vi "Comunicacion_con_Leds.vi"() -> ()   [LabVIEW 2020]
panel:
  in  "Stop":bool
  out "Valor hexadecimal":dbl
  in  "Botón de Contador":bool
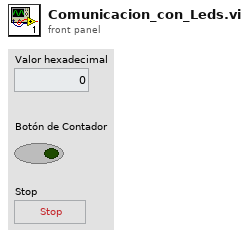
[diagram p1: front panel]
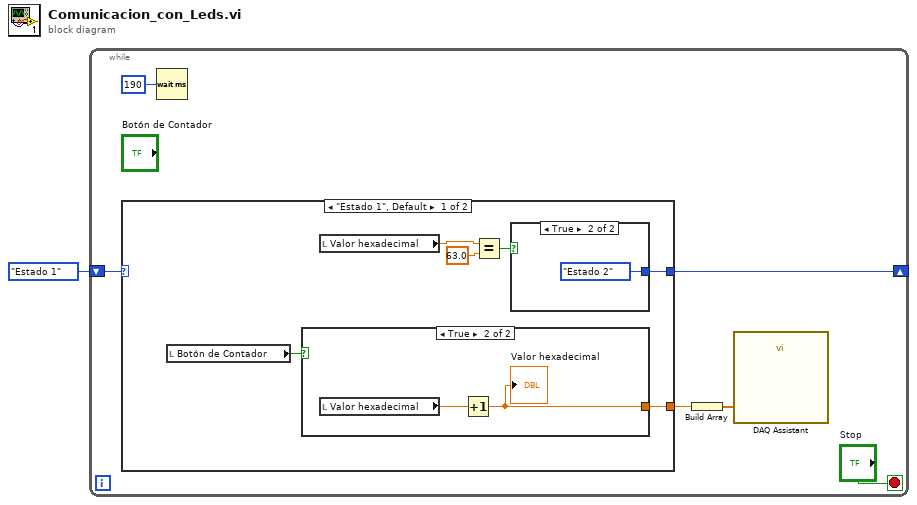
[diagram p0: block diagram]
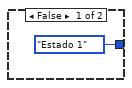
[diagram p2: hidden frame]
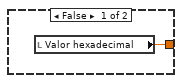
[diagram p3: hidden frame]
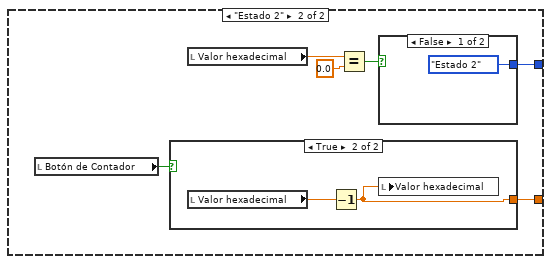
[diagram p4: hidden frame]
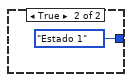
[diagram p5: hidden frame]
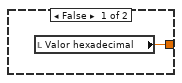
[diagram p6: hidden frame]
diagram:
  n1 = while {
    shift-right: [w5] -> _
    shift-left: enum16{"Estado 1", "Estado 2"}."Estado 1" -> [w6]
    stop <- "Stop" stop-if-true
    n2 = case shown="\"Estado 1\", Default" w6 {
      tunnel: [w13 w24] -> w5
      tunnel: [w11 w23] -> w3
      frame "Estado 1", Default {
        n3 = local read "Botón de Contador"() -> (w12:bool)
        n4 = case shown="True" w12 {
          tunnel: [w16 w18] -> w11
          frame False {
            n5 = local read "Valor hexadecimal"() -> (w16:dbl)
          }
          frame True {
            n6 = local read "Valor hexadecimal"() -> (w17:dbl)
            n7 = Increment(x=w17) -> (x+1=w18:dbl)
            "Valor hexadecimal" <- w18
          }
        }
        n8 = local read "Valor hexadecimal"() -> (w10:dbl)
        n9 = Equal?(x=w10, y=63.0) -> (x = y?=w8:bool)
        n10 = case shown="True" w8 {
          tunnel: [enum16{"Estado 1", "Estado 2"}."Estado 1" enum16{"Estado 1", "Estado 2"}."Estado 2"] -> w13
          frame False {
          }
          frame True {
          }
        }
      }
      frame "Estado 2" {
        n11 = local read "Botón de Contador"() -> (w22:bool)
        n12 = case shown="True" w22 {
          tunnel: [w27 w29] -> w23
          frame False {
            n13 = local read "Valor hexadecimal"() -> (w27:dbl)
          }
          frame True {
            n14 = local read "Valor hexadecimal"() -> (w28:dbl)
            n15 = Decrement(x=w28) -> (x-1=w29:dbl)
            n16 = local write "Valor hexadecimal"(w29) -> ()
          }
        }
        n17 = local read "Valor hexadecimal"() -> (w20:dbl)
        n18 = Equal?(x=w20, y=0.0) -> (x = y?=w19:bool)
        n19 = case shown="False" w19 {
          tunnel: [enum16{"Estado 1", "Estado 2"}."Estado 2" enum16{"Estado 1", "Estado 2"}."Estado 1"] -> w24
          frame False {
          }
          frame True {
          }
        }
      }
    }
    n20 = Wait (ms)(milliseconds to wait=u32 190) -> ()  [unwired: 1 out]
    n21 = Build Array(w3) -> (w2:dbl[])
    n22 = call "DAQ Assistant"("data"=w2) -> ()  [unwired: 17 in, 2 out]
  }
